vi "Launcher.vi"() -> ()   [LabVIEW 2016, in "Test Server Manager.lvlib"]
uses:
  Test Server Manager.lvlib
  WS Test Server/WS Test Server.lvclass
  C:/Program Files (x86)/National Instruments/LabVIEW 2016/vi.lib/ActorFramework/Actor/Actor.lvclass
  WebSocket Actor/WebSocket Server Manager/WebSocket Server Manager.lvclass
  WS Test Server/WS Test Server.lvclass/WS Test Server.ctl
  WS Test Client/WS Test Client.lvclass
  WS Test Server/properties/Write WebSocket Server Manager Enqueuer.vi
  <vilib>/ActorFramework/Actor/Actor.lvclass
panel:
  in  "Number of Clients":i32=1
  out "error out":errorcluster
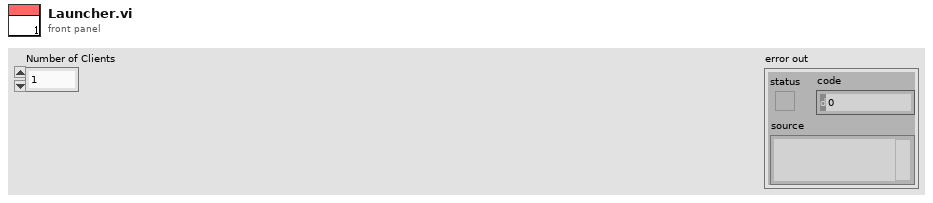
[diagram p1: front panel]
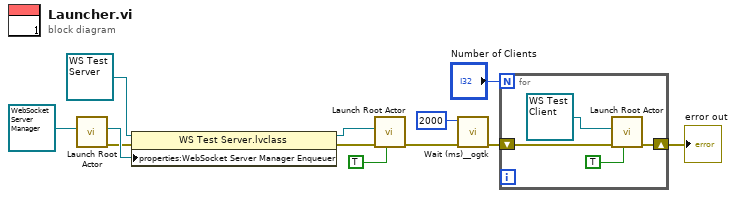
[diagram p0: block diagram]
diagram:
  n1 = call <vilib>:"Launch Root Actor.vi"("Actor"=refnum<class "WebSocket Server Manager.lvclass"> refnum ("WebSocket Actors.lvlib:WebSocket Server Manager.lvclass")) -> ("error out"=w5:errorcluster, "Actor's Enqueuer"=w6:refnum<class "Message Enqueuer.lvclass">)  [unwired: 9 in]
  n2 = property class="WS Test Server.lvclass"(reference=refnum<class "WS Test Server.lvclass"> refnum ("WS Full LabVIEW Test.lvlib:WS Test Server.lvclass"), error in=w5, "properties:WebSocket Server Manager Enqueuer"=w6) -> (reference out=w7:refnum<class "WS Test Server.lvclass">, error out=w4:errorcluster)
  n3 = call <vilib>:"Launch Root Actor.vi"("Open Actor Core front panel? (F)"=TRUE, "error in (no error)"=w4, "Actor"=w7) -> ("error out"=w10:errorcluster)  [unwired: 7 in, 1 out]
  n4 = call <userlib>:"Wait (ms)__ogtk.vi"("error in (no error)"=w10, "milliseconds to wait"=u32 2000) -> ("error out"=w3:errorcluster)  [unwired: 8 in, 1 out]
  n5 = for {
    N: "Number of Clients" -> [_]
    shift-right: [w14] -> w9
    shift-left: w3 -> [w13]
    n6 = call <vilib>:"Launch Root Actor.vi"("Open Actor Core front panel? (F)"=TRUE, "error in (no error)"=w13, "Actor"=refnum<class "WS Test Client.lvclass"> refnum ("WS Full LabVIEW Test.lvlib:WS Test Client.lvclass")) -> ("error out"=w14:errorcluster)  [unwired: 7 in, 1 out]
  }
  "error out" <- w9
